vi "Update VIPB Version.vi"(8 "error in (no error)":errorcluster, 9 "Build Only":bool, 10 "New Version":string, 11 "Full Path":path) -> (0 "error out":errorcluster)   [LabVIEW 2011, in "G CLI VIP.lvlib"]
uses:
  G CLI VIP.lvlib
  <vilib>/JKI/VIPM API/VIPM API_vipm_api.lvlib
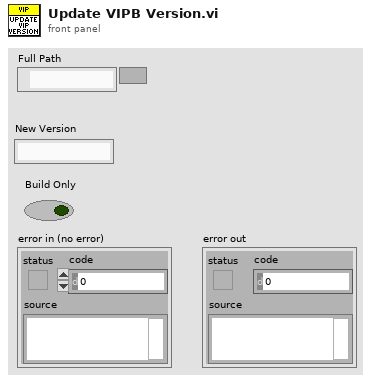
[diagram p1: front panel]
types:
  T1 = typedef "VIPM API_vipm_api.lvlib/VI Package Build Spec Data Cluster_vipm_api.ctl" = cluster{"Package Version":T2, "Product Name":string, "Company Name":string, "Author Name (Person or Company)":string, "Product Homepage (URL)":string, "Legal Copyright":string, "License Agreement Name":string, "Product Description Summary":string, "Product Description":string, "Release Notes - Change Log":string}
  T2 = typedef "VIPM API_vipm_api.lvlib/Version Info Cluster_vipm_api.ctl" = cluster{"major":u32, "minor":u32, "patch":u32, "build":u32}
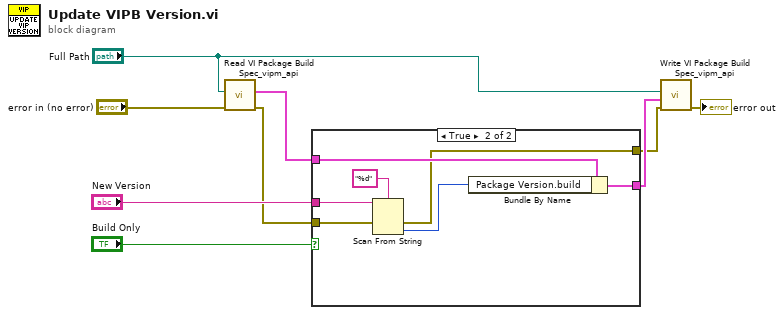
[diagram p0: block diagram]
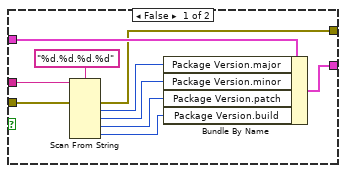
[diagram p2: hidden frame]
diagram:
  n1 = call <vilib>:"Read VI Package Build Spec_vipm_api.vi"("error in (no error)"="error in (no error)", "Path to VIPB File"="Full Path") -> ("error out"=w1:errorcluster, "VI Package Build Spec Data"=w6:T1)  [unwired: 8 in]
  n2 = case shown="True" "Build Only" {
    tunnel: [w19 w26] -> w7
    tunnel: w6 -> [w18 w25]
    tunnel: "New Version" -> [w17 w24]
    tunnel: [w15 w22] -> w2
    tunnel: w1 -> [w14 w21]
    frame False {
      n3 = Scan From String(format string="%d.%d.%d.%d", input string=w17, error in=w14) -> (error out=w15:errorcluster, output 1=w13:i32, output 2=w12:i32, output 3=w11:i32, output 4=w10:i32)  [unwired: 5 in, 2 out]
      n4 = Bundle By Name(cluster=w18, "Package Version.major"=w13, "Package Version.minor"=w12, "Package Version.patch"=w11, "Package Version.build"=w10) -> (w19:T1)
    }
    frame True {
      n5 = Scan From String(format string="%d", input string=w24, error in=w21) -> (error out=w22:errorcluster, output 1=w20:i32)  [unwired: 2 in, 2 out]
      n6 = Bundle By Name(cluster=w25, "Package Version.build"=w20) -> (w26:T1)
    }
  }
  n7 = call <vilib>:"Write VI Package Build Spec_vipm_api.vi"("error in (no error)"=w2, "VI Package Build Spec Data"=w7, "Path to VIPB File"="Full Path") -> ("error out"=→"error out":errorcluster)  [unwired: 8 in]
